vi "Configure Pattern Trigger.vi"(8 "error in (no error)":errorcluster {"code" format="%.0x"}, 9 "trigger level (0.0 V)":dbl caption="Trigger Level (0.0 V)" format="%^.2e", 10 "pattern (\"XXXXXXXXXXXXXXXXXX\")":string="XXXXXXXXXXXXXXXXXX" caption="Pattern (\"XXXXXXXXXXXXXXXXXX\")", 11 "VISA Resource Name":refnum<visa-resource-name>) -> (0 "error out":errorcluster {"code" format="%.0x"}, 3 "VISA Resource Name Out":refnum<visa-resource-name>)   [LabVIEW 2011, in "Agilent 546XX Series.lvlib"]
doc: "This VI configures the trigger level and logical AND combination pattern for the pattern trigger.\n\nNotes: This VI affects instrument behavior only if the trigger type is Pattern. Call the ag546xx Configure Trigger and ag546xx Configure Trigger Coupling VIs to set the trigger type and trigger coupling before calling this VI."
uses:
  Agilent 546XX Series.lvlib
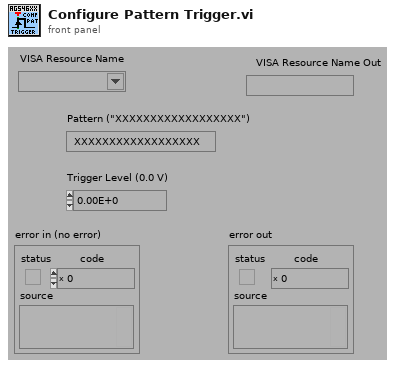
[diagram p1: front panel]
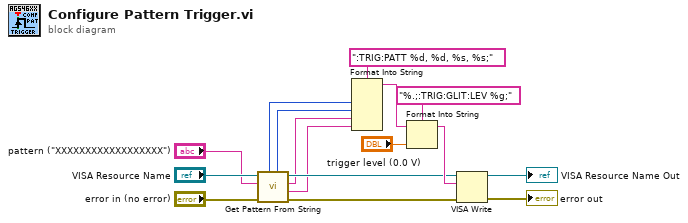
[diagram p0: block diagram]
diagram:
  n1 = call "Get Pattern From String.vi"("error in (no error)"="error in (no error)", "String Pattern (\"XXXXXXXXXXXXXXXXXX\")"="pattern (\"XXXXXXXXXXXXXXXXXX\")", "VISA Resource Name"="VISA Resource Name") -> ("error out"=w6:errorcluster, "Slope"=w1:string, "Edge Source"=w2:string, "VISA Resource Name Out"=w7:refnum<visa-resource-name>, "Mask"=w3:u32, "Pattern Value"=w4:u32)  [unwired: 3 in]
  n2 = Format Into String(format string=":TRIG:PATT %d, %d, %s, %s;", w4, w3, w2, w1) -> (resulting string=w11:string)  [unwired: 2 in, 1 out]
  n3 = Format Into String(format string="%.;:TRIG:GLIT:LEV %g;", initial string=w11, "trigger level (0.0 V)") -> (resulting string=w10:string)  [unwired: 1 in, 1 out]
  n4 = VISA Write(VISA resource name=w7, write buffer=w10, error in (no error)=w6) -> (VISA resource name out=→"VISA Resource Name Out":refnum<visa-resource-name>, error out=→"error out":errorcluster)  [unwired: 1 out]
